vi "Save DataLog.vi"(0 "calculate_doa_data Array":T3[][](array[typedef]), 1 "Data Log Path":path, 2 "append to file? (new file:F)":bool, 5 "calculate_doa_head Array":T2[](array[typedef]), 7 "cal_params":T1[][](array[typedef]), 9 "Amplitude":sgl[][](array[numeric]), 11 "error in (no error)":errorcluster) -> (4 "cal_params_mean":T1[](array[typedef]), 15 "error out":errorcluster)   [LabVIEW 2024]
uses:
  Controls/calculate_doa_struct.ctl
  Controls/ant re&im.ctl
  Controls/Calc Para_int.ctl
  Controls/calculate_doa_head.ctl
  Controls/Calc Para_float.ctl
  <vilib>/Analysis/baseanly.llb/Mean (DBL).vi
  <vilib>/Utility/file.llb/Write Delimited Spreadsheet (string).vi
  <vilib>/Analysis/NI_AALBase.lvlib
panel:
  out "transposed array":string[][](array[string])
  out "Numeric":i32
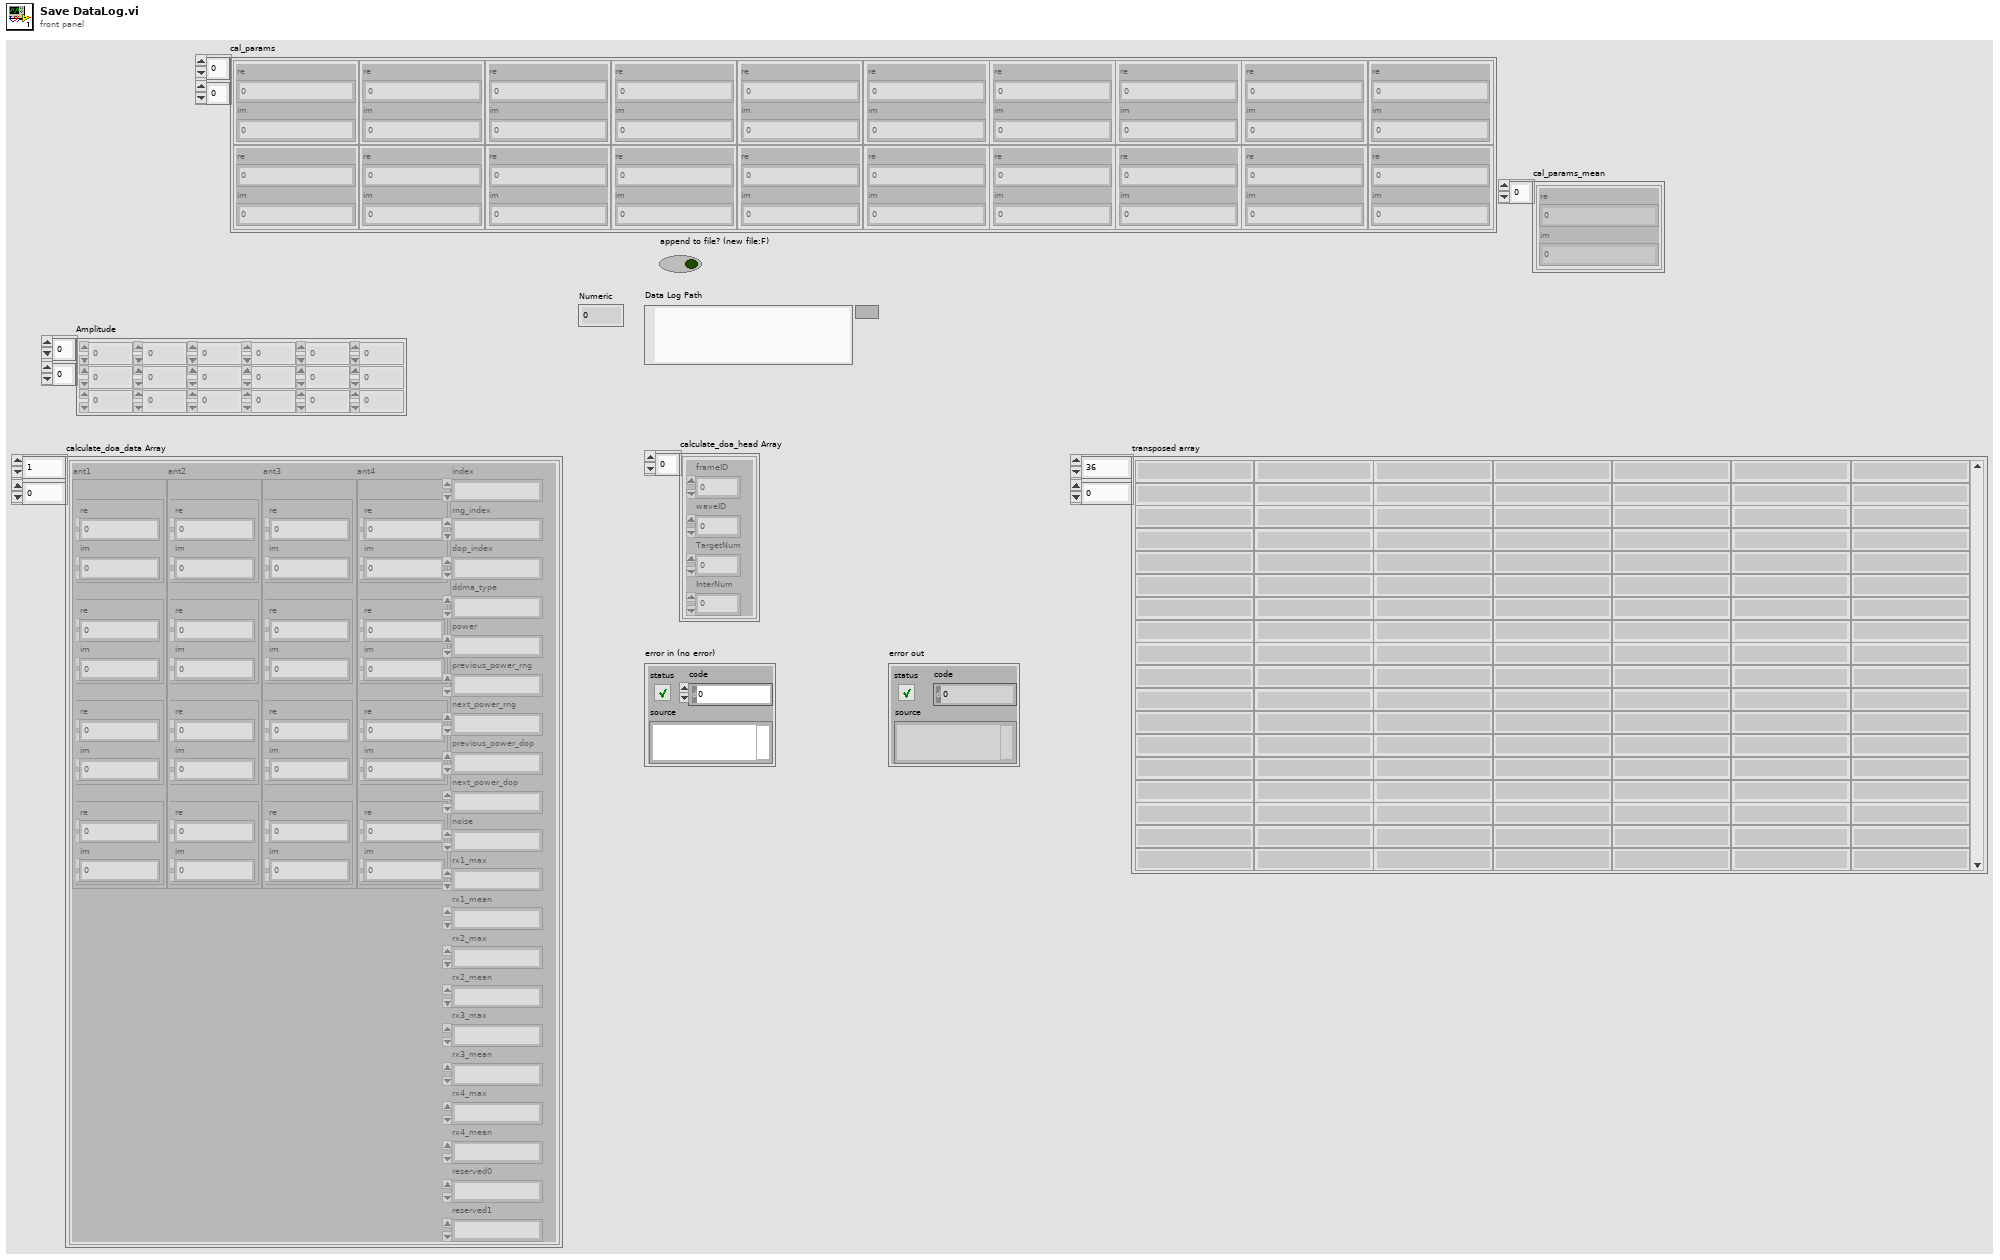
[diagram p1: front panel]
types:
  T1 = typedef "Calc Para_float.ctl" = cluster{"re":sgl, "im":sgl}
  T2 = typedef "calculate_doa_head.ctl" = cluster{"frameID":u16, "waveID":u16, "TargetNum":u16, "InterNum":u16}
  T3 = typedef "calculate_doa_struct.ctl" = cluster{"ant1":T4, "ant2":T4, "ant3":T4, "ant4":T4, "index":u16, "rng_index":u16, "dop_index":u16, "ddma_type":u16, "power":u32, "previous_power_rng":u32, "next_power_rng":u32, "previous_power_dop":u32, "next_power_dop":u32, "noise":u32, "rx1_max":u32, "rx1_mean":u32, "rx2_max":u32, "rx2_mean":u32, "rx3_max":u32, "rx3_mean":u32, "rx4_max":u32, "rx4_mean":u32, "reserved0":u32, "reserved1":u32}
  T4 = typedef "ant re&im.ctl" = cluster{"tx_4":T5, "tx_1":T5, "tx_2":T5, "tx_3":T5}
  T5 = typedef "Calc Para_int.ctl" = cluster{"re":i32, "im":i32}
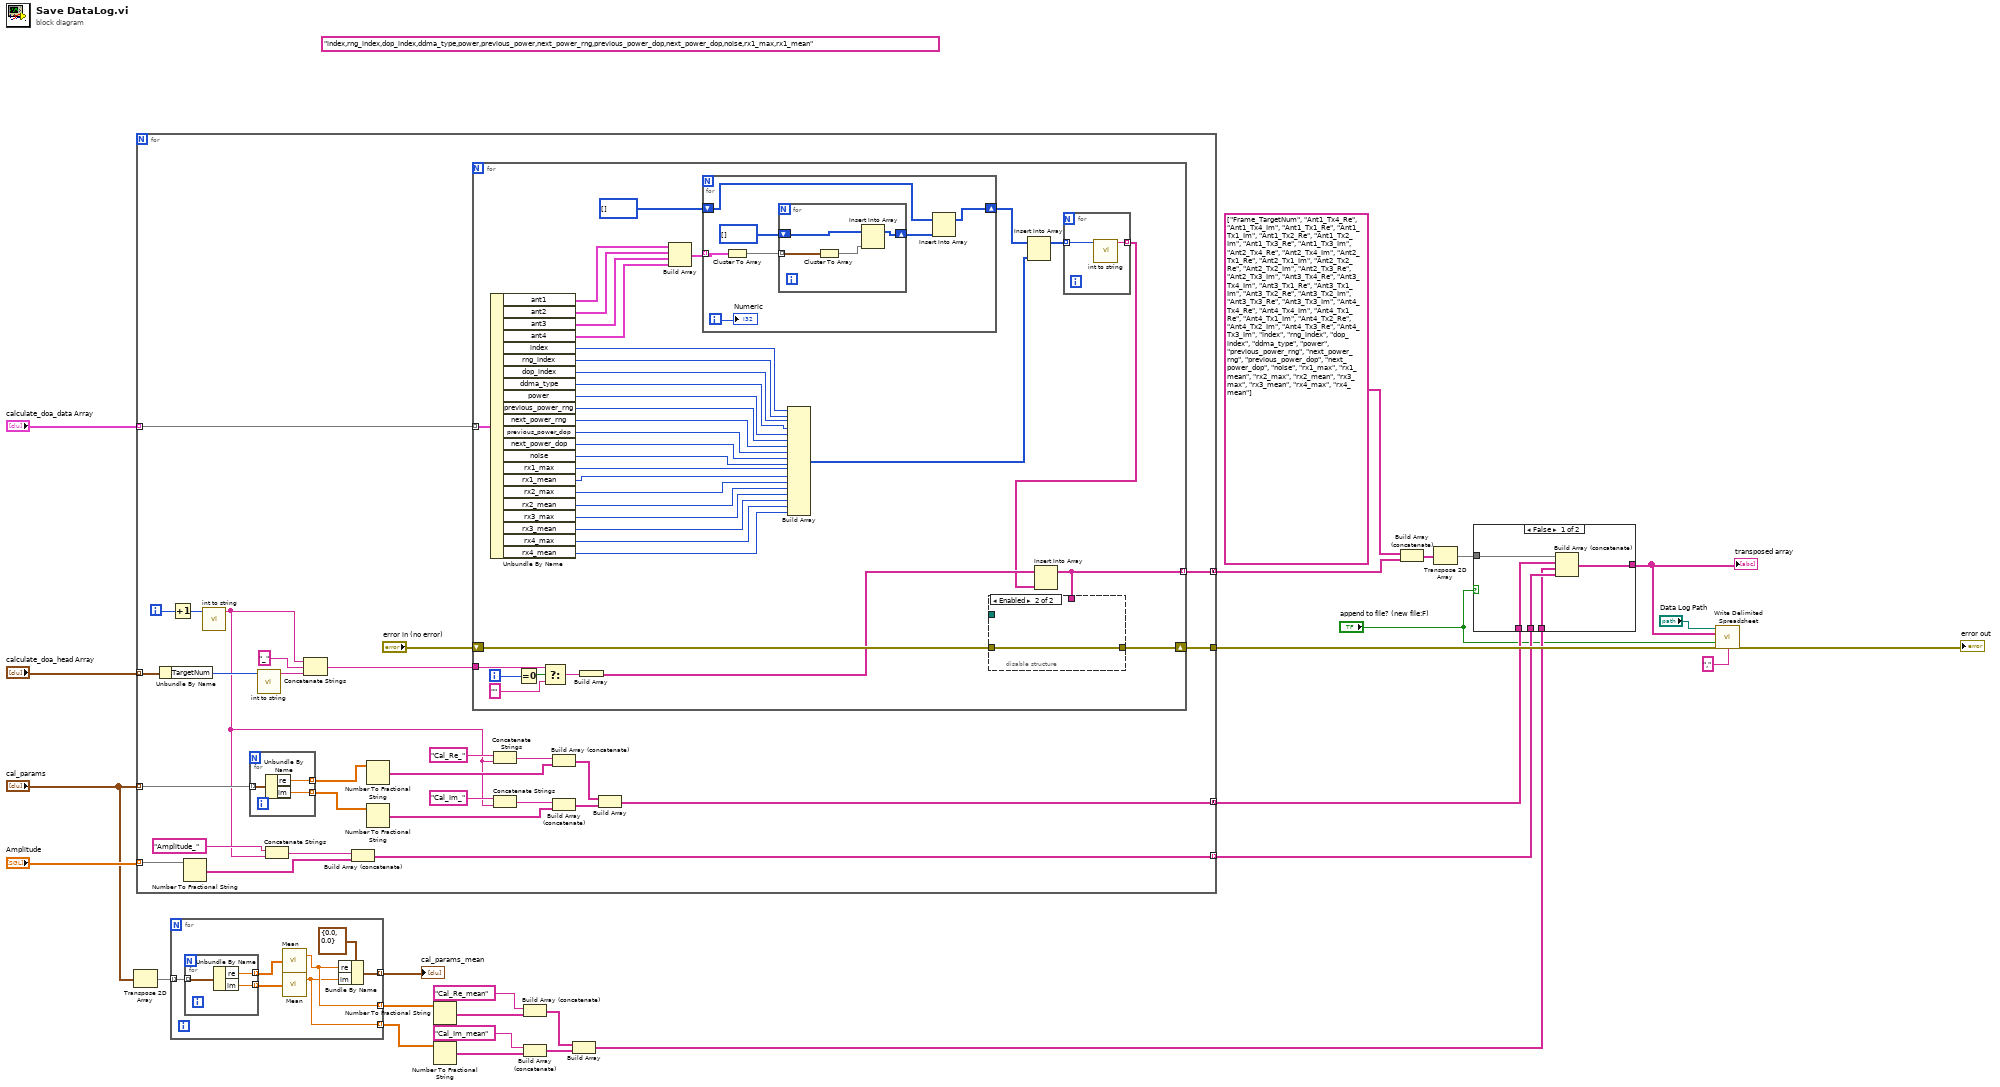
[diagram p0: block diagram]
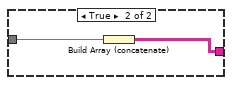
[diagram p2: hidden frame]
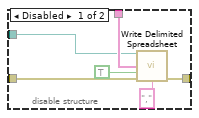
[diagram p3: hidden frame]
diagram:
  (unwired) "index,rng_index,dop_index,ddma_type,power,previous_power,next_power_rng,previous_power_dop,next_power_dop,noise,rx1_max,rx1_mean"
  n1 = Transpose 2D Array(2D array="cal_params") -> (transposed array=w17:T1[][])
  n2 = for {
    tunnel: "calculate_doa_head Array" -> [w53] mode=indexing
    tunnel: "calculate_doa_data Array" -> [w50] mode=indexing
    tunnel: [w47] -> w23 mode=concatenating
    tunnel: [w46] -> w25
    tunnel: "Amplitude" -> [w44] mode=indexing
    tunnel: [w41] -> w6 mode=indexing
    tunnel: "cal_params" -> [w40] mode=indexing
    tunnel: [w28] -> w18 mode=concatenating
    i -> [w51]
    n3 = Unbundle By Name(w53) -> ("TargetNum"=w52:u16)
    n4 = Increment(x=w51) -> (x+1=w49:i32)
    n5 = Number To Fractional String(number=w44) -> (F-format string=w42:string[])  [unwired: 3 in]
    n6 = call "int to string.vi"("number"=w49) -> ("string"=w33:string)  [unwired: 10 in]
    n7 = for {
      tunnel: w40 -> [w59] mode=indexing
      tunnel: [w58] -> w37 mode=indexing
      tunnel: [w57] -> w34 mode=indexing
      n8 = Unbundle By Name(w59) -> ("re"=w58:sgl, "im"=w57:sgl)
    }
    n9 = call "int to string.vi"("number"=w52) -> ("string"=w54:string)  [unwired: 10 in]
    n10 = Concatenate Strings("Amplitude_" ("string"), w33) -> (w43:string)
    n11 = Concatenate Strings(w33, "_" ("string"), w54) -> (w55:string)
    n12 = Build Array (concatenate)(w43, w42) -> (w41:string[])
    n13 = Number To Fractional String(number=w37) -> (F-format string=w35:string[])  [unwired: 3 in]
    n14 = Number To Fractional String(number=w34) -> (F-format string=w32:string[])  [unwired: 3 in]
    n15 = for {
      shift-right: [w96] -> w46
      shift-left: "error in (no error)" -> [w97]
      tunnel: w55 -> [w64]
      tunnel: [w61] -> w47 mode=indexing
      tunnel: w50 -> [w60] mode=indexing
      i -> [w66]
      n16 = Unbundle By Name(w60) -> ("ant1"=w94:T4, "ant2"=w93:T4, "ant3"=w92:T4, "ant4"=w91:T4, "index"=w87:u16, "rng_index"=w86:u16, "dop_index"=w85:u16, "ddma_type"=w84:u16, "power"=w83:u32, "previous_power_rng"=w82:u32, "next_power_rng"=w81:u32, "previous_power_dop"=w80:u32, "next_power_dop"=w79:u32, "noise"=w78:u32, "rx1_max"=w77:u32, "rx1_mean"=w76:u32, "rx2_max"=w75:u32, "rx2_mean"=w74:u32, "rx3_max"=w73:u32, "rx3_mean"=w72:u32, "rx4_max"=w71:u32, "rx4_mean"=w70:u32)
      n17 = Equal To 0?(x=w66) -> (x = 0?=w65:bool)
      n18 = Select(t=w64, s=w65, f="") -> (s? t:f=w63:string)
      n19 = Build Array(w63) -> (w95:string[])
      n20 = Build Array(w94, w93, w92, w91) -> (w90:T4[])
      n21 = for {
        tunnel: w90 -> [w112] mode=indexing
        shift-right: [w108] -> w88
        shift-left: i32[] [] ("array") -> [w110]
        i -> [w107]
        n22 = Cluster To Array(cluster=w112) -> (array=w113:T5[])
        n23 = for {
          tunnel: w113 -> [w117] mode=indexing
          shift-right: [w114] -> w109
          shift-left: i32[] [] ("array") -> [w116]
          n24 = Cluster To Array(cluster=w117) -> (array=w115:i32[])
          n25 = Insert Into Array(array=w116, new element=w115) -> (w114:i32[])  [unwired: 1 in]
        }
        n26 = Insert Into Array(array=w110, new element=w109) -> (w108:i32[])  [unwired: 1 in]
        "Numeric" <- w107
      }
      n27 = Build Array(w87, w86, w85, w84, w83, w82, w81, w80, w79, w78, w77, w76, w75, w74, w73, w72, w71, w70) -> (w69:u32[])
      n28 = Insert Into Array(array=w88, new element=w69) -> (w68:i32[])  [unwired: 1 in]
      n29 = for {
        tunnel: w68 -> [w106] mode=indexing
        tunnel: [w105] -> w67 mode=indexing
        n30 = call "int to string.vi"("number"=w106) -> ("string"=w105:string)  [unwired: 10 in]
      }
      n31 = Insert Into Array(array=w95, new element=w67) -> (w61:string[])  [unwired: 1 in]
      n32 = disable-structure shown="Enabled" {
        disable-tunnel: w97 -> [w103 w104]
        disable-tunnel: [w102 w104] -> w96
        disable-tunnel: w61 -> [w101 _]
        disable-tunnel: _ -> [w98 _]
        frame Disabled {
          n33 = call-poly <vilib>:"Write Delimited Spreadsheet.vi"("file path (dialog if empty)"=w98, "1D data"=w101, "append to file? (new file:F)"=TRUE, "error in (no error)"=w103, "delimiter (\\t)"="," ("delimiter (\\t)")) -> ("error out"=w102:errorcluster)  [unwired: 9 in, 1 out]
        }
        frame Enabled {
        }
      }
    }
    n34 = Concatenate Strings("Cal_Re_" ("string"), w33) -> (w36:string)
    n35 = Concatenate Strings("Cal_Im_" ("string"), w33) -> (w31:string)
    n36 = Build Array (concatenate)(w36, w35) -> (w30:string[])
    n37 = Build Array (concatenate)(w31, w32) -> (w29:string[])
    n38 = Build Array(w30, w29) -> (w28:string[][])
  }
  n39 = for {
    tunnel: w17 -> [w124] mode=indexing
    tunnel: [w120] -> w15 mode=indexing
    tunnel: [w119] -> w8 mode=indexing
    tunnel: [w118] -> w7 mode=indexing
    n40 = for {
      tunnel: w124 -> [w127] mode=indexing
      tunnel: [w126] -> w123 mode=indexing
      tunnel: [w125] -> w122 mode=indexing
      n41 = Unbundle By Name(w127) -> ("re"=w126:sgl, "im"=w125:sgl)
    }
    n42 = call-poly <vilib>:"Mean.vi"("X"=w123) -> ("mean"=w119:dbl)  [unwired: 1 out]
    n43 = call-poly <vilib>:"Mean.vi"("X"=w122) -> ("mean"=w118:dbl)  [unwired: 1 out]
    n44 = Bundle By Name(cluster=T1 {"re"=0.0, "im"=0.0} ("calibration_parameters"), "re"=w119, "im"=w118) -> (w120:T1)
  }
  "cal_params_mean" <- w15
  n45 = Number To Fractional String(number=w8) -> (F-format string=w10:string[])  [unwired: 3 in]
  n46 = Number To Fractional String(number=w7) -> (F-format string=w11:string[])  [unwired: 3 in]
  n47 = Build Array (concatenate)("Cal_Re_mean" ("string"), w10) -> (w13:string[])
  n48 = Build Array (concatenate)("Cal_Im_mean" ("string"), w11) -> (w14:string[])
  n49 = Build Array(w13, w14) -> (w5:string[][])
  n50 = Build Array (concatenate)(string[] ["Frame_TargetNum", "Ant1_Tx4_Re", "Ant1_Tx4_Im", "Ant1_Tx1_Re", "Ant1_Tx1_Im", "Ant1_Tx2_Re", "Ant1_Tx2_Im", "Ant1_Tx3_Re", "Ant1_Tx3_Im", "Ant2_Tx4_Re", "Ant2_Tx4_Im", "Ant2_Tx1_Re", "Ant2_Tx1_Im", "Ant2_Tx2_Re", "Ant2_Tx2_Im", "Ant2_Tx3_Re", "Ant2_Tx3_Im", "Ant3_Tx4_Re", "Ant3_Tx4_Im", "Ant3_Tx1_Re", "Ant3_Tx1_Im", "Ant3_Tx2_Re", "Ant3_Tx2_Im", "Ant3_Tx3_Re", "Ant3_Tx3_Im", "Ant4_Tx4_Re", "Ant4_Tx4_Im", "Ant4_Tx1_Re", "Ant4_Tx1_Im", "Ant4_Tx2_Re", "Ant4_Tx2_Im", "Ant4_Tx3_Re", "Ant4_Tx3_Im", "index", "rng_index", "dop_index", "ddma_type", "power", "previous_power_rng", "next_power_rng", "previous_power_dop", "next_power_dop", "noise", "rx1_max", "rx1_mean", "rx2_max", "rx2_mean", "rx3_max", "rx3_mean", "rx4_max", "rx4_mean"] ("array"), w23) -> (w22:string[][])
  n51 = Transpose 2D Array(2D array=w22) -> (transposed array=w20:string[][])
  n52 = case shown="False" "append to file? (new file:F)" {
    tunnel: w20 -> [w132 w134]
    tunnel: [w131 w133] -> w19
    tunnel: w18 -> [w130 _]
    tunnel: w6 -> [w129 _]
    tunnel: w5 -> [w128 _]
    frame False {
      n53 = Build Array (concatenate)(w132, w130, w128, w129) -> (w131:string[][])
    }
    frame True {
      n54 = Build Array (concatenate)(w134) -> (w133:string[][])
    }
  }
  "transposed array" <- w19
  n55 = call-poly <vilib>:"Write Delimited Spreadsheet.vi"("file path (dialog if empty)"="Data Log Path", "2D data"=w19, "append to file? (new file:F)"="append to file? (new file:F)", "error in (no error)"=w25, "delimiter (\\t)"="," ("delimiter (\\t)")) -> ("error out"=→"error out":errorcluster)  [unwired: 9 in, 1 out]
